vi "Error Code Validation.vi"(9 "Error Name":string, 10 "New Error Code":i32, 11 "Error Codes and Descriptions":string[][](array[string])) -> (3 "Continue":bool)   [LabVIEW 2019, in "Panther Dashboard.lvlib"]
uses:
  Panther Dashboard.lvlib
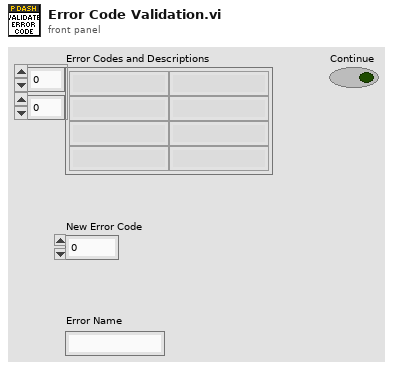
[diagram p1: front panel]
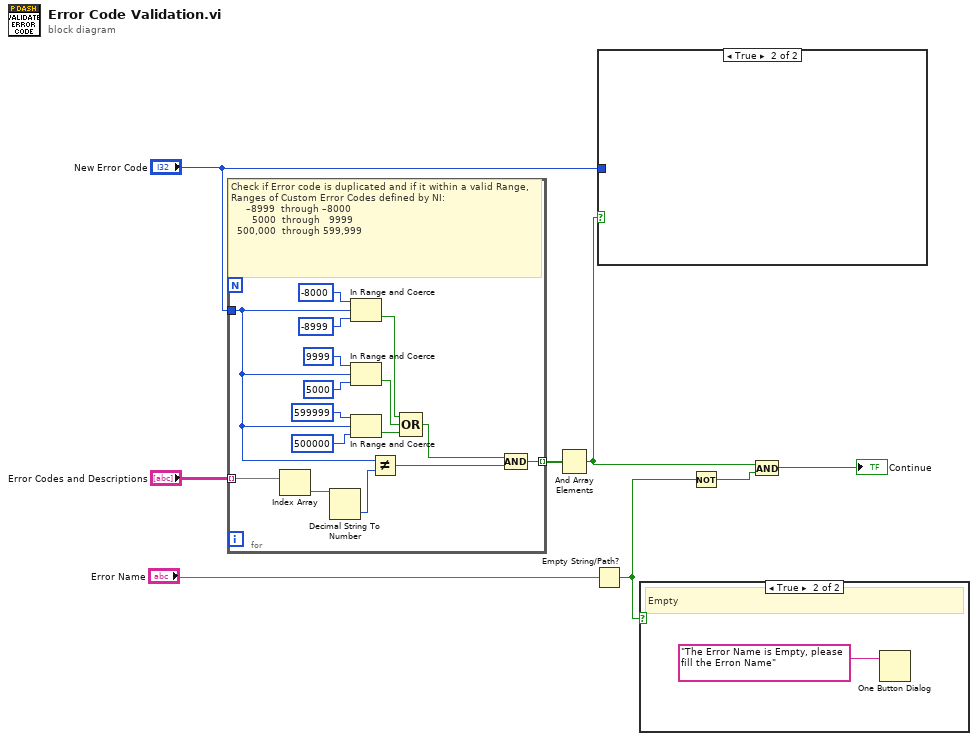
[diagram p0: block diagram]
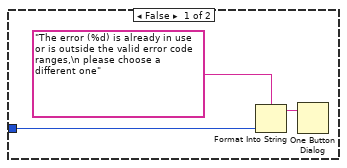
[diagram p3: hidden frame]
diagram:
  n1 = for {
    tunnel: "Error Codes and Descriptions" -> [w11] mode=indexing
    tunnel: "New Error Code" -> [w18]
    tunnel: [w17] -> w8 mode=indexing
    # "Check if Error code is duplicated and if it within a valid Range,\nRanges of Custom Error Codes defined by NI:\n     –8999  through –8000\n       5000  through   9999\n  500,000  through 599,999"
    n2 = Index Array(array=w11) -> (element=w10:string)  [unwired: 1 in]
    n3 = Decimal String To Number(string=w10) -> (number=w9:i32)  [unwired: 2 in, 1 out]
    n4 = In Range and Coerce(upper limit=-8000, x=w18, lower limit=-8999 ("upper limit")) -> (In Range?=w16:bool)  [unwired: 1 out]
    n5 = In Range and Coerce(upper limit=9999, x=w18, lower limit=5000 ("upper limit")) -> (In Range?=w15:bool)  [unwired: 1 out]
    n6 = In Range and Coerce(upper limit=599999, x=w18, lower limit=500000 ("upper limit")) -> (In Range?=w14:bool)  [unwired: 1 out]
    n7 = Not Equal?(x=w18, y=w9) -> (x != y?=w13:bool)
    n8 = Compound Arithmetic op=OR(w16, w15, w14) -> (w12:bool)
    n9 = Compound Arithmetic op=AND(w12, w13) -> (w17:bool)
  }
  n10 = And Array Elements(Boolean array=w8) -> (logical AND=w4:bool)
  n11 = Empty String/Path?(string/path="Error Name") -> (empty?=w1:bool)
  n12 = case shown="True" w4 {
    tunnel: "New Error Code" -> [w26 _]
    frame False {
      n13 = Format Into String(format string="The error (%d) is already in use or is outside the valid error code ranges,\n please choose a different one", w26) -> (resulting string=w27:string)  [unwired: 2 in, 1 out]
      n14 = One Button Dialog(message=w27) -> ()  [unwired: 1 in, 1 out]
    }
    frame True {
    }
  }
  n15 = case shown="True" w1 {
    frame False {
      # "Non Empty"
    }
    frame True {
      # "Empty"
      n16 = One Button Dialog(message="The Error Name is Empty, please fill the Erron Name" ("format string")) -> ()  [unwired: 1 in, 1 out]
    }
  }
  n17 = Not(x=w1) -> (.not. x?=w2:bool)
  n18 = And(x=w4, y=w2) -> (x .and. y?=→"Continue":bool)
